vi "03 - Exemple - AsyncSum.vi"() -> ()   [LabVIEW 2016]
uses:
  Library/DemoSkeleton/DemoSkeleton.lvlib
panel:
  in  "B":i32=2
  in  "A":i32=1
  out "Sum":i64
  # "+"
  # "="
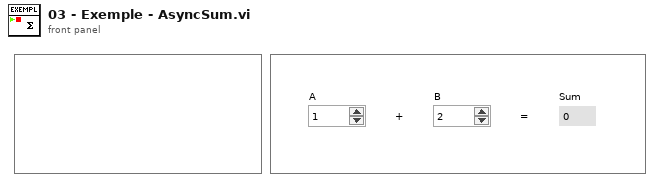
[diagram p1: front panel]
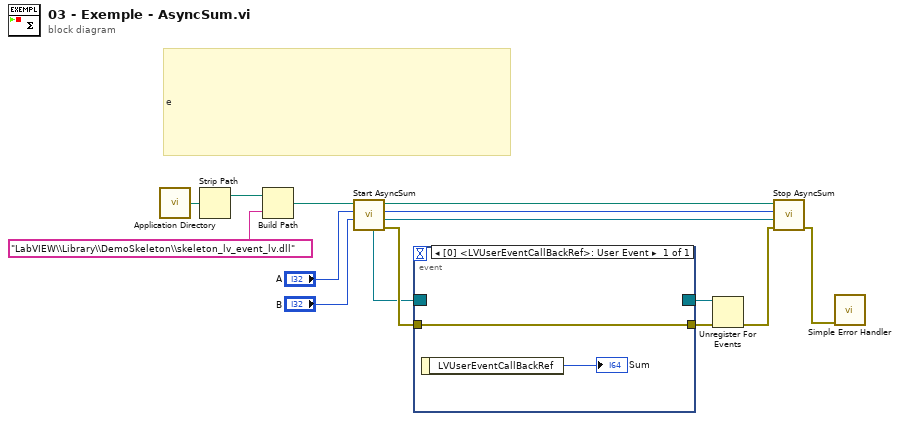
[diagram p0: block diagram]
diagram:
  # "e"
  n1 = call <vilib>:"Application Directory.vi"() -> ("Application Directory"=w4:path)
  n2 = Strip Path(path=w4) -> (stripped path=w3:path)  [unwired: 1 out]
  n3 = Build Path(base path=w3, name or relative path="LabVIEW\\Library\\DemoSkeleton\\skeleton_lv_event_lv.dll") -> (appended path=w2:path)
  n4 = call "Start AsyncSum.vi"("B"="B", "A"="A", "path in"=w2) -> ("error out"=w13:errorcluster, "LVUserEvent CallBack Reference"=w7:refnum<user-event>, "Handle"=w11:u64, "dup path"=w12:path, "AsyncSum Event Register"=w8:refnum<event-registration>)  [unwired: 4 in]
  n5 = event shown="[0] <LVUserEventCallBackRef>: User Event" {
    selector: w8 -> [_]
    dyn-events: [_] -> w15
    timeout: _ -> [_]
    tunnel: w13 -> [w17]
    tunnel: [w17] -> w14
    event User Event {
      n6 = event-data() -> ("LVUserEventCallBackRef"=→"Sum":i64)  [unwired: 1 in]
    }
  }
  n7 = Unregister For Events(event registration refnum=w15, error in=w14) -> (error out=w10:errorcluster)
  n8 = call "Stop AsyncSum.vi"("error in (no error)"=w10, "LVUserEventCallBackRef"=w7, "Handle"=w11, "path in"=w12) -> ("error out"=w9:errorcluster)  [unwired: 6 in, 1 out]
  n9 = call <vilib>:"Simple Error Handler.vi"("error in (no error)"=w9) -> ()  [unwired: 4 in, 5 out]
